vi "Initialize.vi"(8 "error in (no error)":errorcluster, 9 "Password":string, 10 "Username":string, 11 "Server-URL":string="http://159.89.102.81") -> (0 "error out":errorcluster, 3 "ByteGSWebAPI-V0 out":refnum<class "ByteGSWebAPI-V0.lvclass">)   [LabVIEW 2019, in "ByteGSWebAPI.lvlib" / "ByteGSWebAPI-V0.lvclass"]
uses:
  ByteGSWebAPI-V0.lvclass
  ByteGSWebAPI-V0.lvclass/ByteGSWebAPI-V0.ctl
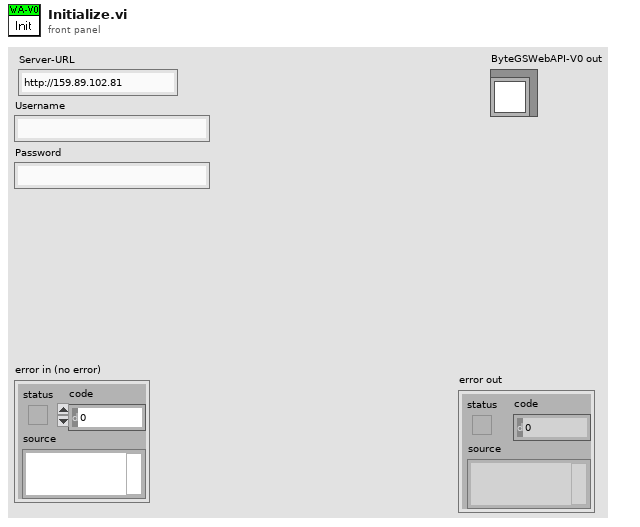
[diagram p1: front panel]
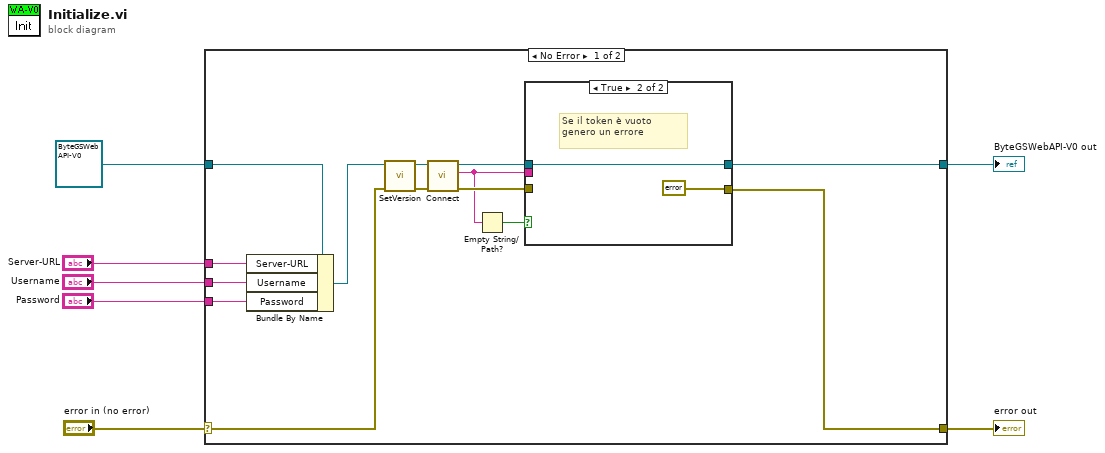
[diagram p0: block diagram]
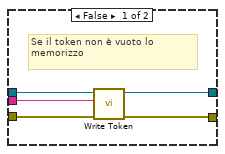
[diagram p2: hidden frame]
diagram:
  n1 = case shown="No Error" "error in (no error)" {
    selector: "error in (no error)" -> [w16 w30]
    tunnel: [w9 w30] -> w6
    tunnel: [w11 w29] -> w4
    tunnel: refnum<class "ByteGSWebAPI-V0.lvclass"> refnum ("ByteGSWebAPI-V0 in") -> [w21 w29]
    tunnel: "Server-URL" -> [w20 _]
    tunnel: "Username" -> [w19 _]
    tunnel: "Password" -> [w18 _]
    frame No Error {
      n2 = Bundle By Name(cluster=w21, "Server-URL"=w20, "Username"=w19, "Password"=w18) -> (w17:refnum<class "ByteGSWebAPI-V0.lvclass">)
      n3 = call-dynamic "SetVersion.vi"("error in (no error)"=w16, "ByteGSWebAPI-V0 in"=w17) -> ("error out"=w14:errorcluster, "ByteGSWebAPI-V0 out"=w15:refnum<class "ByteGSWebAPI-V0.lvclass">)  [unwired: 8 in]
      n4 = call-dynamic "Connect.vi"("error in (no error)"=w14, "ByteGSWebAPI-V0 in"=w15) -> ("error out"=w10:errorcluster, "token"=w8:string, "ByteGSWebAPI-V0 out"=w12:refnum<class "ByteGSWebAPI-V0.lvclass">)  [unwired: 5 in, 2 out]
      n5 = Empty String/Path?(string/path=w8) -> (empty?=w13:bool)
      n6 = case shown="True" w13 {
        tunnel: w12 -> [w24 w28]
        tunnel: [w23 w28] -> w11
        tunnel: w10 -> [w25 _]
        tunnel: [w26 errorcluster {"status"=TRUE, "code"=0, "source"="Empty Token"} ("error in (no error)")] -> w9
        tunnel: w8 -> [w22 _]
        frame False {
          # "Se il token non è vuoto lo\nmemorizzo"
          n7 = call-dynamic "Write Token.vi"("error in (no error)"=w25, "Token"=w22, "ByteGSWebAPI-V0 in"=w24) -> ("error out"=w26:errorcluster, "ByteGSWebAPI-V0 out"=w23:refnum<class "ByteGSWebAPI-V0.lvclass">)  [unwired: 7 in]
        }
        frame True {
          # "Se il token è vuoto \ngenero un errore"
        }
      }
    }
    frame Error {
    }
  }
  "error out" <- w6
  "ByteGSWebAPI-V0 out" <- w4
